vi "Set_trigger.vi"(5 "Auto_trigger_ms":i16, 6 "Direction":i16, 7 "Threshold":i16, 8 "error in (no error)":errorcluster, 9 "Delay":i16, 10 "Source":i16, 11 "Handle":i16) -> (0 "error out":errorcluster, 3 "return type":i16)   [LabVIEW 2023]
uses:
  ps2000.dll
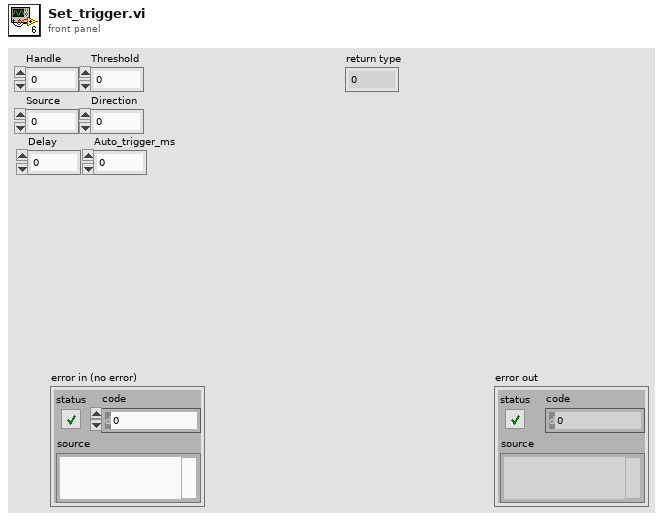
[diagram p1: front panel]
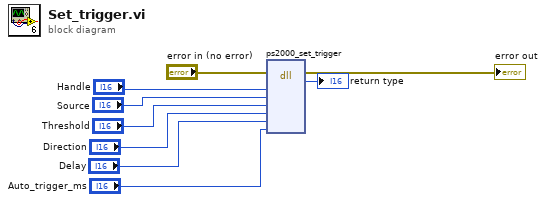
[diagram p0: block diagram]
diagram:
  n1 = dll-call lib="C:/Users/cesar/Desktop/Ps2000 libreria/PS2000.dll" fn="ps2000_set_trigger"(error in="error in (no error)", "handle"="Handle", "source"="Source", "threshold"="Threshold", "direction"="Direction", "delay"="Delay", "auto_trigger_ms"="Auto_trigger_ms") -> (error out=→"error out":errorcluster, "return type"=→"return type":i16)  [unwired: 8 in, 1 out]
